vi "LC_model_management.vi"() -> ()   [LabVIEW 2016]
uses:
  LC_BESS_global.vi
panel:
  out "appended array":dbl[](array[numeric])
  out "x":dbl[][](array[numeric])
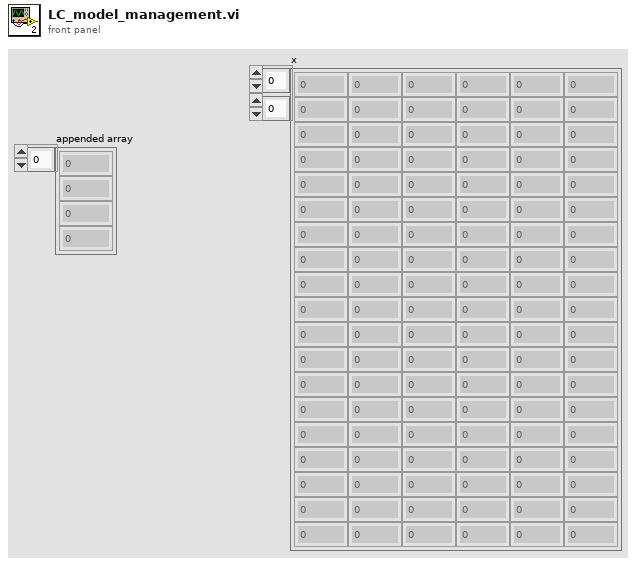
[diagram p1: front panel]
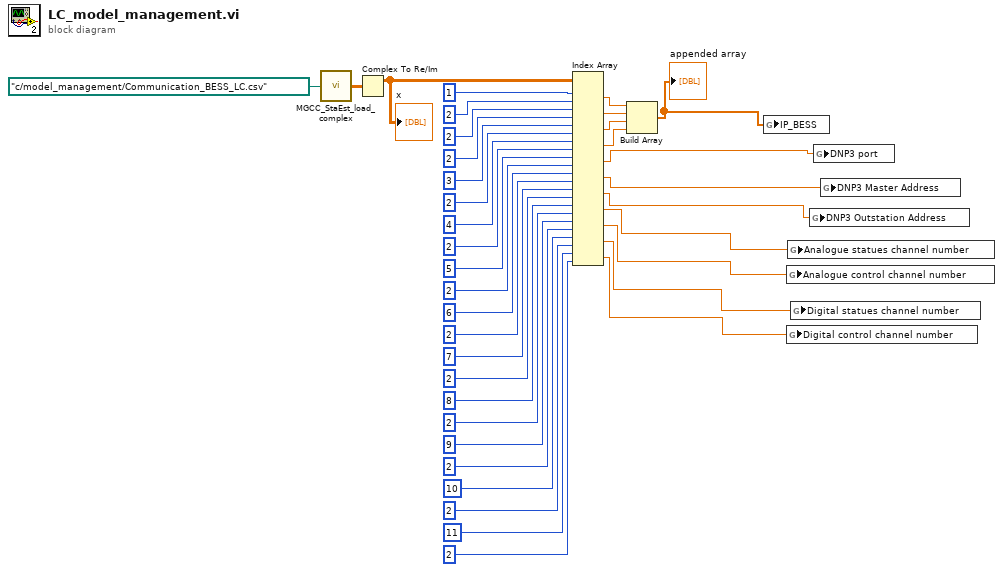
[diagram p0: block diagram]
diagram:
  n1 = call "MGCC_StaEst_load_complex.vi"("file path (dialog if empty)"=path "c:/model_management/Communication_BESS_LC.csv" ("file path (use dialog)")) -> ("Array 13"=w24:cdb[][])
  n2 = Complex To Re/Im(x + iy=w24) -> (x=w23:dbl[][])  [unwired: 1 out]
  "x" <- w23
  n3 = Index Array(array=w23, index (row) #1=1 ("index (row)"), index (col) #1=2 ("disabled index (col)"), index (row) #2=2 ("index (row)"), index (col) #2=2 ("disabled index (col)"), index (row) #3=3 ("index (row)"), index (col) #3=2 ("disabled index (col)"), index (row) #4=4 ("index (row)"), index (col) #4=2 ("disabled index (col)"), index (row) #5=5 ("index (row)"), index (col) #5=2 ("disabled index (col)"), index (row) #6=6 ("index (row)"), index (col) #6=2 ("disabled index (col)"), index (row) #7=7 ("index (row)"), index (col) #7=2 ("disabled index (col)"), index (row) #8=8 ("index (row)"), index (col) #8=2 ("disabled index (col)"), index (row) #9=9 ("index (row)"), index (col) #9=2 ("disabled index (col)"), index (row) #10=10 ("index (row)"), index (col) #10=2 ("disabled index (col)"), index (row) #11=11 ("index (row)"), index (col) #11=2 ("disabled index (col)")) -> (element #1=w34:dbl, element #2=w27:dbl, element #3=w26:dbl, element #4=w25:dbl, element #5=w7:dbl, element #6=w6:dbl, element #7=w5:dbl, element #8=w4:dbl, element #9=w3:dbl, element #10=w2:dbl, element #11=w1:dbl)
  n4 = Build Array(w34, w27, w26, w25) -> (w8:dbl[])
  "appended array" <- w8
  n5 = global write "LC_BESS_global.vi" "IP_BESS"(w8) -> ()
  n6 = global write "LC_BESS_global.vi" "Analogue control channel number"(w3) -> ()
  n7 = global write "LC_BESS_global.vi" "Digital control channel number"(w1) -> ()
  n8 = global write "LC_BESS_global.vi" "Analogue statues channel number"(w4) -> ()
  n9 = global write "LC_BESS_global.vi" "Digital statues channel number"(w2) -> ()
  n10 = global write "LC_BESS_global.vi" "DNP3 Outstation Address"(w5) -> ()
  n11 = global write "LC_BESS_global.vi" "DNP3 port"(w7) -> ()
  n12 = global write "LC_BESS_global.vi" "DNP3 Master Address"(w6) -> ()
